vi "Nano-drive-lambda.vi"(5 "Set this axis?":cluster{"X":bool, "Y":bool, "Z":bool}, 6 "Z (um)":ext format="%.4f", 7 "Y (um)":ext format="%.4f", 9 "Numeric":i32, 10 "X (um)":ext format="%.4f") -> ()   [LabVIEW 2014]
doc: "Moves the Mad City piezo stage by a fixed amount in x, y, and z"
uses:
  Program Files (x86)/Gelles Lab Software/Madlib.dll
panel:
  out "z readout":dbl
  out "y readout":dbl
  out "x readout":dbl
  # "Specific for Mad City USB controller"
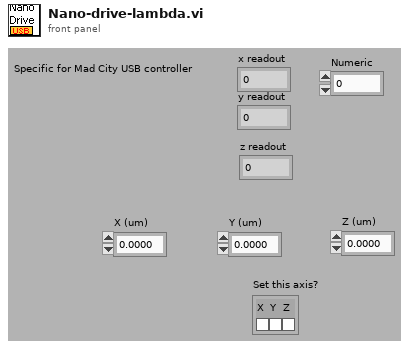
[diagram p1: front panel]
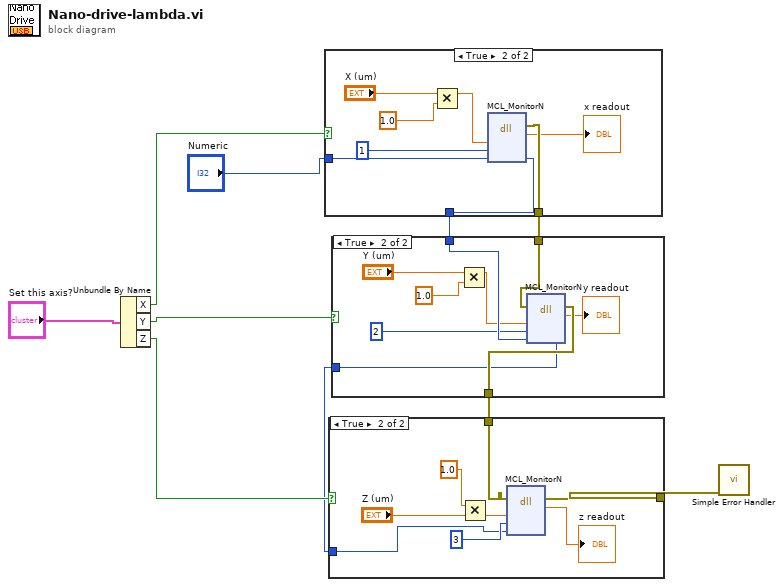
[diagram p0: block diagram]
diagram:
  n1 = Unbundle By Name("Set this axis?") -> ("X"=w9:bool, "Y"=w8:bool, "Z"=w7:bool)
  n2 = case shown="True" w9 {
    tunnel: [_ w19] -> w6
    tunnel: "Numeric" -> [w11 w16]
    tunnel: [w11 w15] -> w3
    frame False {
    }
    frame True {
      n3 = Multiply(x="X (um)", y=1.0) -> (x*y=w13:ext)
      n4 = dll-call lib="C:/Program Files (x86)/Gelles Lab Software/MADLib.dll" fn="MCL_MonitorN"("position"=w13, "axis"=1, "handle"=w16) -> (error out=w19:errorcluster, "return type"=→"x readout":dbl, "handle"=w15:i32)  [unwired: 5 in, 1 out]
    }
  }
  n5 = case shown="True" w8 {
    tunnel: w6 -> [w21 w30]
    tunnel: [w21 w29] -> w5
    tunnel: w3 -> [w20 w27]
    tunnel: [w20 w25] -> w2
    frame False {
    }
    frame True {
      n6 = Multiply(x="Y (um)", y=1.0) -> (x*y=w23:ext)
      n7 = dll-call lib="C:/Program Files (x86)/Gelles Lab Software/MADLib.dll" fn="MCL_MonitorN"(error in=w30, "position"=w23, "axis"=2, "handle"=w27) -> (error out=w29:errorcluster, "return type"=→"y readout":dbl, "handle"=w25:i32)  [unwired: 4 in, 1 out]
    }
  }
  n8 = case shown="True" w7 {
    tunnel: w5 -> [w31 w38]
    tunnel: [w31 w39] -> w4
    tunnel: w2 -> [_ w35]
    frame False {
    }
    frame True {
      n9 = Multiply(x=1.0, y="Z (um)") -> (x*y=w33:ext)
      n10 = dll-call lib="C:/Program Files (x86)/Gelles Lab Software/MADLib.dll" fn="MCL_MonitorN"(error in=w38, "position"=w33, "axis"=3, "handle"=w35) -> (error out=w39:errorcluster, "return type"=→"z readout":dbl)  [unwired: 5 in, 1 out]
    }
  }
  n11 = call <vilib>:"Simple Error Handler.vi"("error in (no error)"=w4) -> ()  [unwired: 1 in, 8 out]
